vi "Instances check days.vi"(8 "Dates in":timestamp[](array[timestamp]), 11 "Array in":string[](array[string])) -> (0 "Dates undelivered":timestamp[](array[timestamp]), 3 "Array out":string[](array[string]))   [LabVIEW 2015]
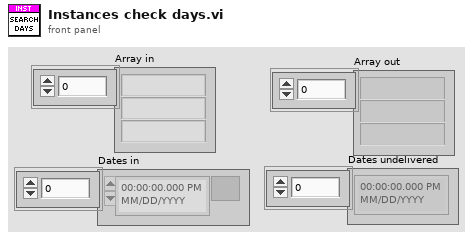
[diagram p1: front panel]
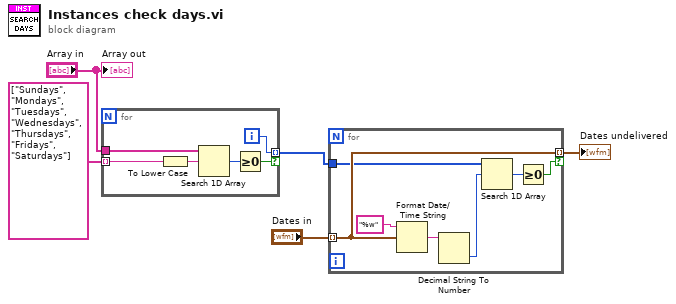
[diagram p0: block diagram]
diagram:
  n1 = for {
    tunnel: "Array in" -> [w11]
    tunnel: string[] ["Sundays", "Mondays", "Tuesdays", "Wednesdays", "Thursdays", "Fridays", "Saturdays"] -> [w10] mode=indexing
    tunnel: [w7] -> w3 mode=indexing if=w6
    i -> [w7]
    n2 = To Lower Case(string=w10) -> (all lower case string=w9:string)
    n3 = Search 1D Array(1D array=w11, element=w9) -> (index of element=w8:i32)  [unwired: 1 in]
    n4 = Greater Or Equal To 0?(x=w8) -> (x >= 0?=w6:bool)
  }
  n5 = for {
    tunnel: "Dates in" -> [w16] mode=indexing
    tunnel: w3 -> [w15]
    tunnel: [w16] -> w5 mode=indexing if=w12
    n6 = Format Date/Time String(time format string (%c)="%w", seconds (now)=w16) -> (date/time string=w17:string)  [unwired: 1 in]
    n7 = Decimal String To Number(string=w17) -> (number=w14:i32)  [unwired: 2 in, 1 out]
    n8 = Search 1D Array(1D array=w15, element=w14) -> (index of element=w13:i32)  [unwired: 1 in]
    n9 = Greater Or Equal To 0?(x=w13) -> (x >= 0?=w12:bool)
  }
  "Dates undelivered" <- w5
  "Array out" <- "Array in"
